vi "CallVI.ml.vi"(0 "n":i32, 1 "mlp":u64, 2 "MathLink Dll":path) -> ()   [LabVIEW 2014]
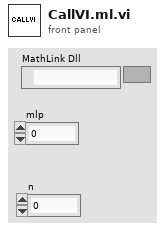
[diagram p1: front panel]
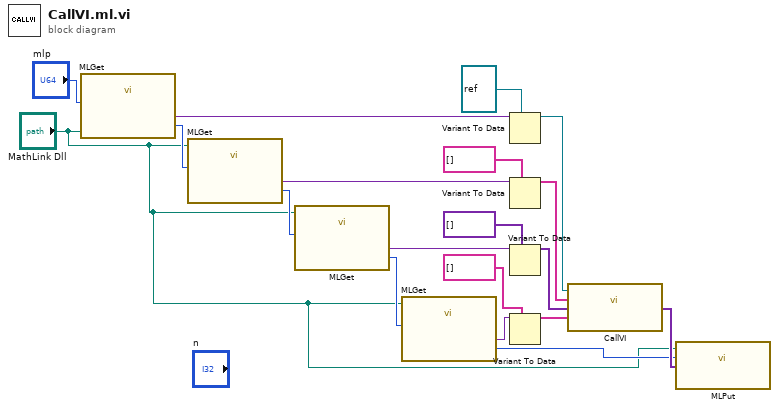
[diagram p0: block diagram]
diagram:
  n1 = call "MLGet.vi"("mlp in"="mlp", "MathLink Dll"="MathLink Dll") -> ("Variant"=w9:variant, "mlp out"=w11:u64)  [unwired: 1 in, 4 out]
  n2 = call "MLGet.vi"("mlp in"=w11, "MathLink Dll"="MathLink Dll") -> ("Variant"=w10:variant, "mlp out"=w8:u64)  [unwired: 1 in, 4 out]
  n3 = call "MLGet.vi"("mlp in"=w8, "MathLink Dll"="MathLink Dll") -> ("Variant"=w7:variant, "mlp out"=w6:u64)  [unwired: 1 in, 4 out]
  n4 = call "MLGet.vi"("mlp in"=w6, "MathLink Dll"="MathLink Dll") -> ("Variant"=w5:variant, "mlp out"=w3:u64)  [unwired: 1 in, 4 out]
  n5 = Variant To Data(type=refnum<vi> refnum ("vi reference"), Variant=w9) -> (data=w16:refnum<vi>)  [unwired: 1 in, 1 out]
  n6 = Variant To Data(type=string[] [] ("Input Names"), Variant=w10) -> (data=w17:string[])  [unwired: 1 in, 1 out]
  n7 = Variant To Data(type=variant[] [] ("Input Values"), Variant=w7) -> (data=w18:variant[])  [unwired: 1 in, 1 out]
  n8 = Variant To Data(type=string[] [] ("Input Names"), Variant=w5) -> (data=w19:string[])  [unwired: 1 in, 1 out]
  n9 = call "CallVI.vi"("Output Names"=w19, "Input Values"=w18, "Input Names"=w17, "VI"=w16) -> ("Output Values"=w4:variant[])
  n10 = call "MLPut.vi"("Variant"=w4, "mlp in"=w3, "MathLink Dll"="MathLink Dll") -> ()  [unwired: 1 in, 1 out]
